vi "T3AWG Config Panel.vi"(8 "error in (no error)":errorcluster, 11 "t3awg in":T5={"VISA"="", "use ext ref"=FALSE, "ext ref [Hz]"=0.0, "load Z"=enum."High Z", "ramdac max n"=0, "noise dither [V]"=0.0, "t3awg fs rules"=[], "channels"=0, "ramdac min n"=0, "channel list"=[], "gen resl [Vpp]"=0.0, "wave data format"=enum."Binary"} {"t3awg fs rules"."fs-step [Hz]" format="%#_6p"; "t3awg fs rules"."fs-max [Hz]" format="%#_6p"; "t3awg fs rules"."for f0 <" format="%#_6p"; "t3awg fs rules"."fs-min [Hz]" format="%#_6p"}) -> (0 "error out":errorcluster, 3 "t3awg out":T5={"VISA"="", "use ext ref"=FALSE, "ext ref [Hz]"=0.0, "load Z"=enum."High Z", "ramdac max n"=0, "noise dither [V]"=0.0, "t3awg fs rules"=[], "channels"=0, "ramdac min n"=0, "channel list"=[], "gen resl [Vpp]"=0.0, "wave data format"=enum."Binary"} {"t3awg fs rules"."fs-step [Hz]" format="%#_6p"; "t3awg fs rules"."fs-max [Hz]" format="%#_6p"; "t3awg fs rules"."for f0 <" format="%#_6p"; "t3awg fs rules"."fs-min [Hz]" format="%#_6p"})   [LabVIEW 2020, in "Active Technologies AWG3000.lvlib"]
uses:
  Active Technologies AWG3000.lvlib
  T3AWG Session.ctl
  T3AWG Load Z.ctl
  fgen_ramdac_fs_rules.ctl
  T3AWG Channel.ctl
panel:
  in  "btn test":bool
  in  "wave data format":T1=enum."Binary" caption="Waveform transfer format"
  in  "gen amp resl [Vpp]":dbl caption="Generator amp resolution [Vpp]" format="%#_6p"
  in  "btn default chn":bool
  in  "Channels":T2[](array[typedef]) caption="Channels (Fixed = T: constant level, F: variable level)" {"A [V]:" format="%#_6p"}
  in  "btn default":bool
  in  "VISA":refnum<visa-resource-name>
  in  "btn ok":bool
  in  "ramdac min n":i32 caption="Minimum RAMDAC samples" format="%.0p"
  in  "noise dither [V]":dbl caption="Noise dithering level [V]" format="%#_6p"
  in  "ramdac max n":i32 caption="Maximum RAMDAC samples" format="%.0p"
  in  "load Z":T3 caption="Output loading"
  in  "ext ref [Hz]":dbl caption="External ref. clock [Hz]" format="%#_6p"
  in  "use ext ref":bool caption="Use external ref clock"
  in  "fs rules":T4[](array[typedef]) caption="Sampling rate selection rules" {"fs-step [Hz]" format="%#_6p"; "fs-max [Hz]" format="%#_6p"; "for f0 <" format="%#_6p"; "fs-min [Hz]" format="%#_6p"}
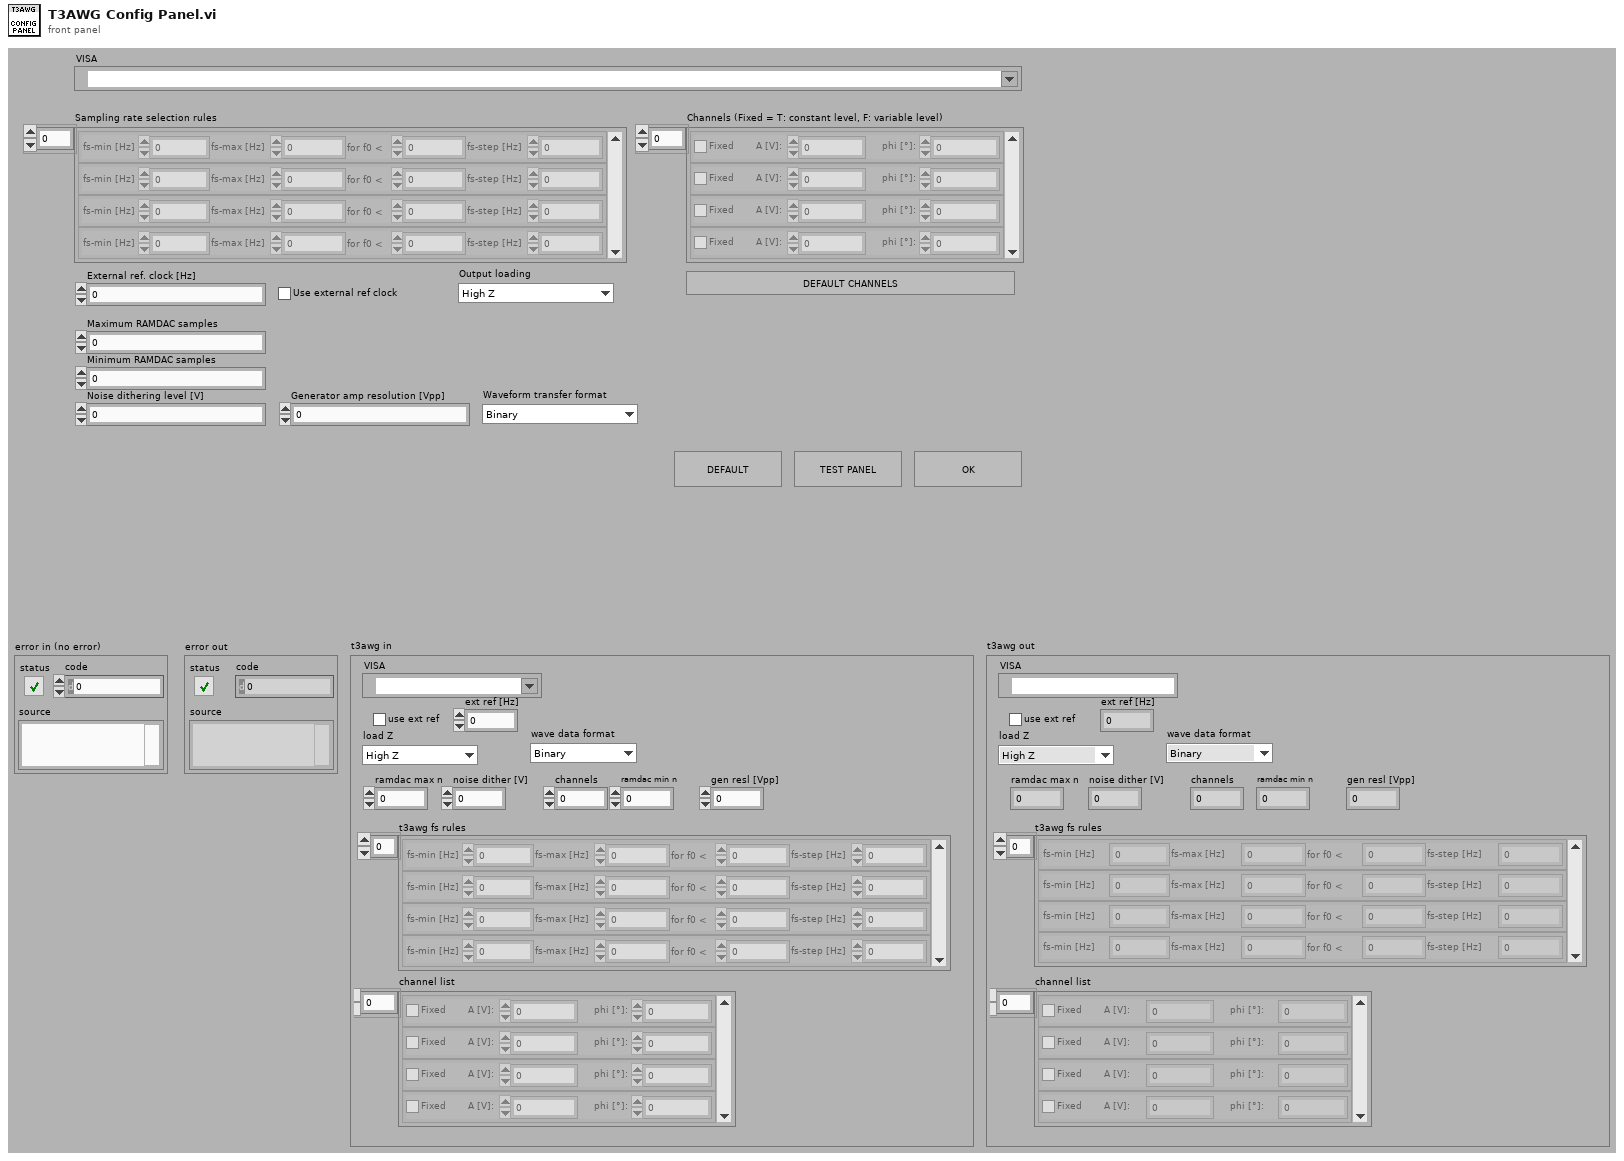
[diagram p1: front panel]
types:
  T1 = typedef "Active Technologies AWG3000.lvlib/T3AWG Wave Format" = enum16{"Text", "Binary"}
  T2 = typedef "Active Technologies AWG3000.lvlib/T3AWG Channel.ctl" = cluster{"Fixed":bool, "A [V]:":dbl, "phi [°]:":dbl}
  T3 = typedef "Active Technologies AWG3000.lvlib/T3AWG Load Z.ctl" = enum16{"High Z", "50 Ohm"}
  T4 = typedef "Active Technologies AWG3000.lvlib/fgen_ramdac_fs_rules.ctl" = cluster{"fs-min [Hz]":dbl, "fs-max [Hz]":dbl, "for f0 < ":dbl, "fs-step [Hz]":dbl}
  T5 = typedef "Active Technologies AWG3000.lvlib/T3AWG Session.ctl" = cluster{"VISA":refnum<visa-resource-name>, "use ext ref":bool, "ext ref [Hz]":dbl, "load Z":T3, "ramdac max n":i32, "noise dither [V]":dbl, "t3awg fs rules":T4[], "channels":i32, "ramdac min n":i32, "channel list":T2[], "gen resl [Vpp]":dbl, "wave data format":T1}
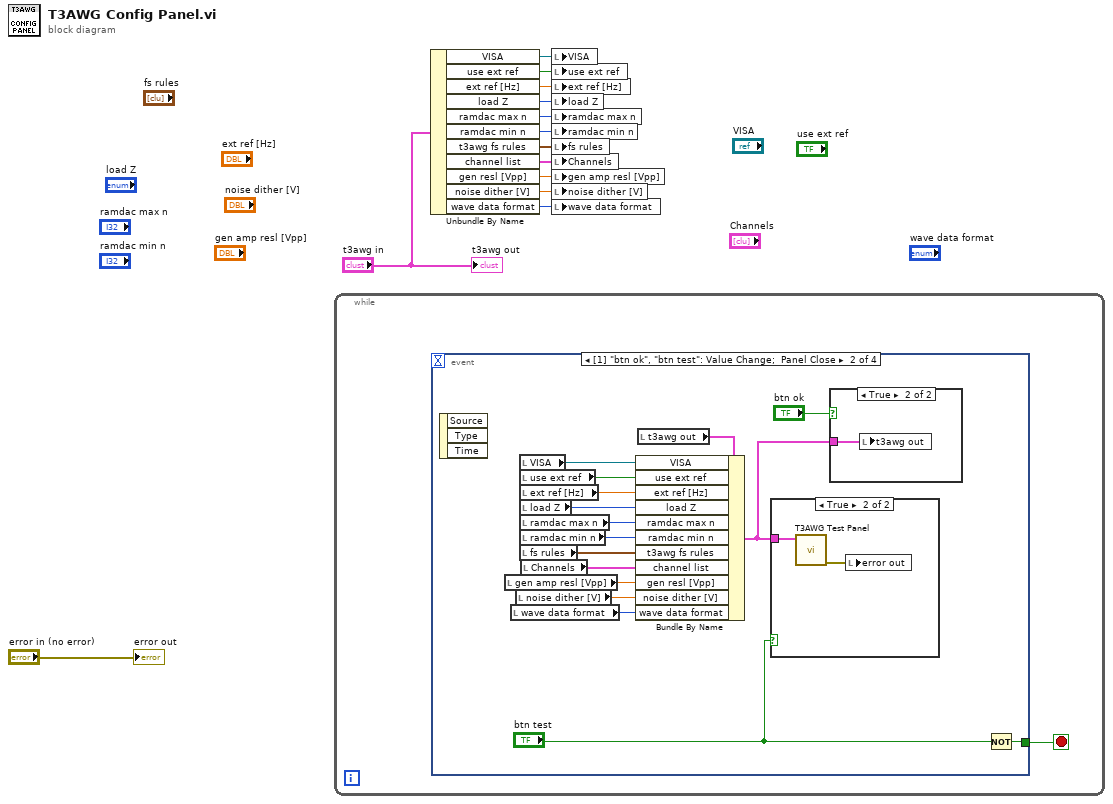
[diagram p0: block diagram]
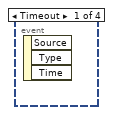
[diagram p2: hidden frame]
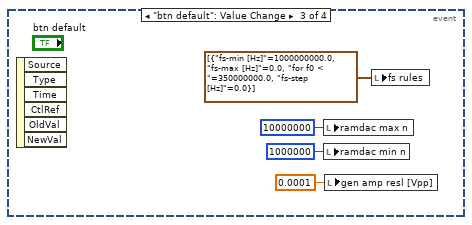
[diagram p5: hidden frame]
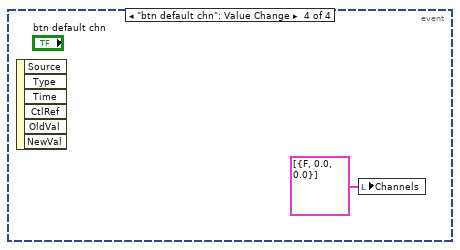
[diagram p6: hidden frame]
diagram:
  n1 = while {
    stop <- w14 stop-if-true
    n2 = event shown="[1] \"btn ok\", \"btn test\": Value Change;  Panel Close" {
      selector: _ -> [_ _ _ _]
      dyn-events: _ -> [_ _ _ _]
      timeout: _ -> [_ _ _ _]
      tunnel: [_ w18 _ _] -> w14
      event Timeout {
        n3 = event-data() -> ()  [unwired: 1 in, 3 out]
      }
      event "btn ok", "btn test": Value Change; Panel Close {
        n4 = event-data() -> ()  [unwired: 1 in, 3 out]
        n5 = local read "gen amp resl [Vpp]"() -> (w21:dbl)
        n6 = local read "wave data format"() -> (w19:T1)
        n7 = local read "noise dither [V]"() -> (w20:dbl)
        n8 = local read "VISA"() -> (w29:refnum<visa-resource-name>)
        n9 = local read "use ext ref"() -> (w28:bool)
        n10 = local read "ext ref [Hz]"() -> (w27:dbl)
        n11 = local read "load Z"() -> (w26:T3)
        n12 = local read "ramdac max n"() -> (w25:i32)
        n13 = local read "ramdac min n"() -> (w24:i32)
        n14 = local read "fs rules"() -> (w23:T4[])
        n15 = local read "Channels"() -> (w22:T2[])
        n16 = local read "t3awg out"() -> (w30:T5)
        n17 = Bundle By Name(cluster=w30, "VISA"=w29, "use ext ref"=w28, "ext ref [Hz]"=w27, "load Z"=w26, "ramdac max n"=w25, "ramdac min n"=w24, "t3awg fs rules"=w23, "channel list"=w22, "gen resl [Vpp]"=w21, "noise dither [V]"=w20, "wave data format"=w19) -> (w15:T5)
        n18 = case shown="True" "btn test" {
          tunnel: w15 -> [_ w33]
          frame False {
          }
          frame True {
            n19 = call "T3AWG Test Panel.vi"("t3awg"=w33) -> ("error out"=w32:errorcluster)  [unwired: 9 in, 1 out]
            n20 = local write "error out"(w32) -> ()
          }
        }
        n21 = case shown="True" "btn ok" {
          tunnel: w15 -> [_ w31]
          frame False {
          }
          frame True {
            n22 = local write "t3awg out"(w31) -> ()
          }
        }
        n23 = Not(x="btn test") -> (.not. x?=w18:bool)
      }
      event "btn default": Value Change {
        n24 = event-data() -> ()  [unwired: 1 in, 6 out]
        n25 = local write "ramdac max n"(10000000 ("ramdac max n")) -> ()
        n26 = local write "ramdac min n"(1000000 ("ramdac min n")) -> ()
        n27 = local write "gen amp resl [Vpp]"(0.0001 ("gen amp resl [Vpp]")) -> ()
        n28 = local write "fs rules"(T4[] [{"fs-min [Hz]"=1000000000.0, "fs-max [Hz]"=0.0, "for f0 < "=350000000.0, "fs-step [Hz]"=0.0}] ("fs rules")) -> ()
      }
      event "btn default chn": Value Change {
        n29 = event-data() -> ()  [unwired: 1 in, 6 out]
        n30 = local write "Channels"(T2[] [{"Fixed"=FALSE, "A [V]:"=0.0, "phi [°]:"=0.0}] ("Channels")) -> ()
      }
    }
  }
  n31 = Unbundle By Name("t3awg in") -> ("VISA"=w11:refnum<visa-resource-name>, "use ext ref"=w10:bool, "ext ref [Hz]"=w9:dbl, "load Z"=w8:T3, "ramdac max n"=w7:i32, "ramdac min n"=w6:i32, "t3awg fs rules"=w5:T4[], "channel list"=w4:T2[], "gen resl [Vpp]"=w3:dbl, "noise dither [V]"=w2:dbl, "wave data format"=w1:T1)
  n32 = local write "VISA"(w11) -> ()
  n33 = local write "use ext ref"(w10) -> ()
  n34 = local write "ext ref [Hz]"(w9) -> ()
  n35 = local write "load Z"(w8) -> ()
  n36 = local write "ramdac max n"(w7) -> ()
  n37 = local write "ramdac min n"(w6) -> ()
  n38 = local write "fs rules"(w5) -> ()
  n39 = local write "Channels"(w4) -> ()
  n40 = local write "gen amp resl [Vpp]"(w3) -> ()
  n41 = local write "noise dither [V]"(w2) -> ()
  n42 = local write "wave data format"(w1) -> ()
  "error out" <- "error in (no error)"
  "t3awg out" <- "t3awg in"
